vi "VCS Clear Fault.vi"(8 "error in (no error)":errorcluster, 11 "axis in":cluster{"keyHandle":u32, "nodeId":u16}={"keyHandle"=0, "nodeId"=1}) -> (0 "error out":errorcluster, 3 "axis out":cluster{"keyHandle":u32, "nodeId":u16}={"keyHandle"=0, "nodeId"=1})   [LabVIEW 2019]
doc: "<B>VCS Clear Fault</B> changes device from fault state to disable state."
uses:
  <instrlib>/Maxon EPOS/maxon EPOS/Resources/EposCmd.dll
  <instrlib>/Maxon EPOS/maxon EPOS/Resources/EposCmd64.dll
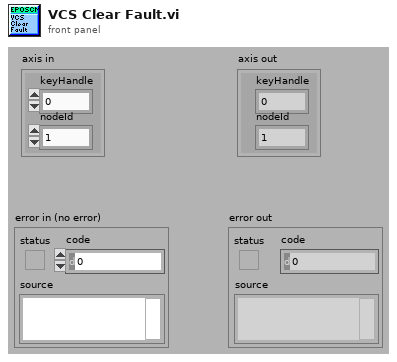
[diagram p1: front panel]
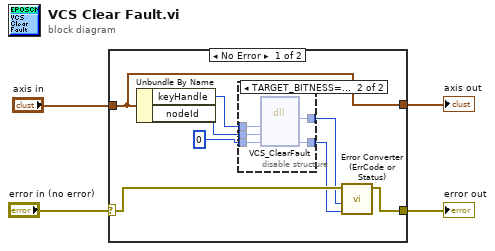
[diagram p0: block diagram]
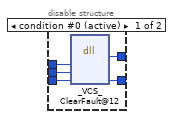
[diagram p2: hidden frame]
diagram:
  n1 = case shown="No Error" "error in (no error)" {
    selector: "error in (no error)" -> [w8 w24]
    tunnel: [w7 w24] -> w3
    tunnel: "axis in" -> [w9 w23]
    tunnel: [w9 w23] -> w1
    frame No Error {
      n2 = Unbundle By Name(w9) -> ("keyHandle"=w12:u32, "nodeId"=w11:u16)
      n3 = disable-structure shown="TARGET_BITNESS==64" {
        disable-tunnel: w12 -> [w17 w22]
        disable-tunnel: w11 -> [w16 w21]
        disable-tunnel: u32 0 ("pErrorCode") -> [w15 w20]
        disable-tunnel: [w14 w19] -> w6
        disable-tunnel: [w13 w18] -> w5
        frame condition #0 (active) {
          n4 = dll-call lib="C:/Program Files (x86)/National Instruments/LabVIEW 2019/instr.lib/Maxon EPOS/maxon EPOS/Resources/EposCmd.*" fn="_VCS_ClearFault@12"("KeyHandle"=w17, "NodeId"=w16, "pErrorCode"=w15) -> (w14:i32, "pErrorCode"=w13:u32)  [unwired: 5 in, 2 out]
        }
        frame condition #1 {
          n5 = dll-call lib="C:/setup/Resources/EposCmd64.*" fn="VCS_ClearFault" ("EposCmd.dll:_VCS_ClearFault@12")("KeyHandle"=w22, "NodeId"=w21, "pErrorCode"=w20) -> ("Rückgabetyp"=w19:i32, "pErrorCode"=w18:u32)  [unwired: 5 in, 2 out]
        }
      }
      n6 = call <instrlib>:"Error Converter (ErrCode or Status).vi"("error code"=w5, "return type"=w6, "error in (no error)"=w8) -> ("error out"=w7:errorcluster)  [unwired: 7 in]
    }
    frame Error {
    }
  }
  "error out" <- w3
  "axis out" <- w1
